vi "Dashboard Main.vi"() -> ()   [LabVIEW 2014]
uses:
  <vilib>/event_ctls.llb/eventvkey.ctl
  <vilib>/Rock Robotics/WPI/Dashboard/WPI_DashboardLogging Global.vi
  <vilib>/Rock Robotics/Network Tables/SD Read Number.vi
  <vilib>/Rock Robotics/Network Tables/SD Read Boolean.vi
  <vilib>/Rock Robotics/Network Tables/SD Write Number.vi
  <vilib>/Rock Robotics/Network Tables/SD Read String.vi
  <vilib>/Utility/config.llb/Write Key (String).vi
  <vilib>/Utility/config.llb/Write Key (I32).vi
  <vilib>/Utility/config.llb/NI_LVConfig.lvlib
panel:
  in  "TCP":refnum<k5>
  in  "Rec Mode":enum32{"Stop", "Record", "Playback"}(radio)
  in  "Vision":u16(ring) items=["Camera Off", "USB Camera SW", "USB Camera HW", "IP Camera"]
  out "Camera IP":string
  out "Image Message":string="Timeout in Camera Communications"
  in  "Dashboard Tab":T1(tab)
  in  "Camera Guide Position":dbl(slide) scale=0.0..320.0
  in  "Camera Settings":T2={"Frame Rate"=30, "Compression"=30, "Size"=1} {"Frame Rate" scale=1.0..30.0; "Size" items=["640x480", "320x240", "160x120"]}
  out "MotorChart R":cluster{"Numeric":dbl, "Numeric":dbl}(graph)
  out "MotorChart L":T3(graph)
  out "MotorSliders R":cluster{"MotorSlide1":dbl, "MotorSlide2":dbl} {"MotorSlide2" scale=-1.0..1.0 scale format="%#_2e"; "MotorSlide1" scale=-1.0..1.0 scale format="%#_2e"}
  out "MotorSliders L":T4 {"MotorSlide4 2" scale=0.0..14.0 scale format="%#_2e"; "MotorSlide2" scale=-1.0..1.0 scale format="%#_2e"; "MotorSlide1" scale=-1.0..1.0 scale format="%#_2e"}
  out "JS1 Z":dbl(slide) scale=-1.0..1.0 scale format="%#_2e"
  out "JS1 Graph":cluster{"X":dbl, "Y":dbl}[](graph)
  out "JS1 Buttons":T5
  out "JS2 Z":dbl(slide) scale=-1.0..1.0 scale format="%#_2e"
  out "JS2 Graph":cluster{"X":dbl, "Y":dbl}[](graph)
  out "JS2 Buttons":T5
  out "Mode":T6(ring)=enum."Auto Disabled"
  in  "DB Camera Config":bool
  out "fps":dbl format="%#.1g"
  out "Mbps":dbl format="%#.1g"
  out "Mbps 2":bool
  out "Current Auto":dbl
  out "Auto/String 3":string caption="DB/String 3"
  out "Auto/String 2":string caption="DB/String 2"
  out "Auto/String 1":string caption="DB/String 1"
  out "Auto/String 0":string caption="Auto"
  out "Can\n  Auto\n  Stack":bool
  out "PID State":T7(ring)
  in  "Training Mode Threshold":dbl=0.8
  out "Drive Mode":bool
  out "Gyro":dbl(knob) scale=0.0..360.0
  in  "Halo Sensitivity":dbl=0.7 min=0.0 max=1.0 step=0.01 format="%.2f"
  out "Encoder Left":dbl
  out "Encoder Right":dbl
  out "Training Enabled":bool
  out "Auto Stack State":T8(ring)
  out "Gripper":bool
  out "Gripper 2":bool
  in  "Test Slider":dbl(slide) scale=0.0..100.0 scale format="%#_3g"
  in  "On/Off":bool caption="Solenoid"
  in  "Test Name":u16(ring) items=["Select the test to run...", "Example Test", "-------------------------------", "List of tests is built in robot code.", "Replace with your own automated tests."]
  in  "Test Tree":string(tree)
  in  "Motor":cluster{"Value":dbl, "Enable":bool} {"Value" scale=-1.0..1.0 scale format="%#_3g"}
  out "Progress":T9 {"Test Progress" scale=0.0..100.0}
  in  "Rev/Fwd":cluster{"Forward":bool, "Reverse":bool}
  in  "Test Ring":u16(ring) items=["Monochrome", "Color"]
  in  "Listbox":i32(listbox)
  out "Tree":string(tree)
  out "Camera Image":T10(plugin-control)
  out "Boolean":bool
  # "Left"
  # "Front"
  # "Right"
  # "Battery"
  # "0 - TOTE+CONTAINER\n1 - DRIVESTRAIGHT FROM STARTING AREA\n2 - DRIVESTRAIGHT FROM VOLDEMORT\n3 - 2 CONTAINER + LEFT TURN\n4 - 2 CONTAINER + RIGHT TURN\n5 - STOP_ALL\n6 - TAPE MEASURE"
  # "Hold BACK button on \nJoystick 1 to switch"
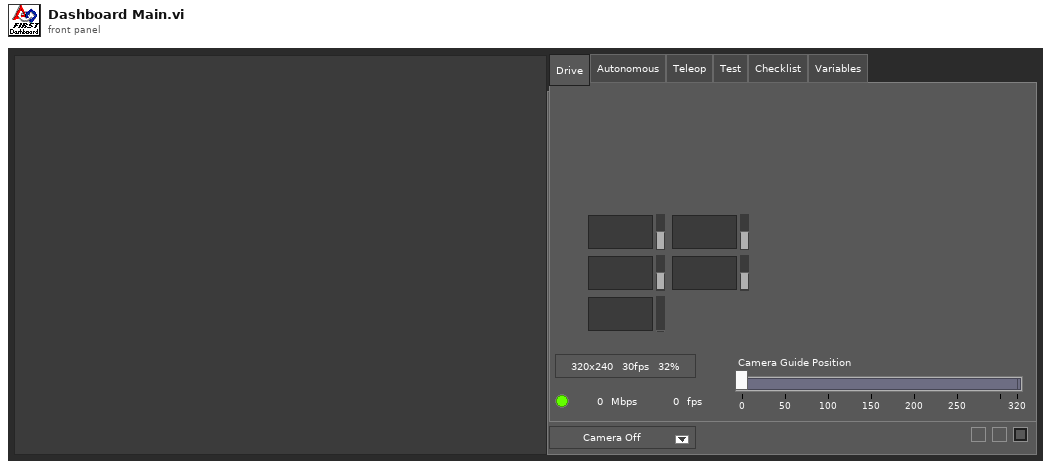
[diagram p1: front panel]
types:
  T1 = enum32{"Drive", "Autonomous", "Teleop", "Test", "Checklist", "Variables"}
  T2 = cluster{"Frame Rate":i32, "Compression":i32, "Size":u16}
  T3 = cluster{"Numeric":dbl, "Numeric":dbl, "Battery V":dbl}
  T4 = cluster{"MotorSlide1":dbl, "MotorSlide2":dbl, "MotorSlide4 2":dbl}
  T5 = cluster{bool, bool, bool, bool, bool, bool, bool, bool, bool, bool, bool, bool}
  T6 = enum8{"Tele-Op Disabled", "Tele-Op Enabled", "Auto Disabled", "Auto Enabled", "Test Disabled", "Test Enabled", "Disconnected", "No Code", "E-Stop"}
  T7 = enum16{"ResetForward", "ResetBack", "PIDControl", "ManualControl", "ZeroEncoderAndTarget", "AutoStack"}
  T8 = enum16{"Disabled", "Initialize", "CalcNewTarget", "Moving", "OpenArm", "CloseArm", "Reset"}
  T9 = cluster{"Test Progress":u8, "Test Progress Text":string}
  T10 = typedef "IMAQ Image.ctl" = refnum<image>
  T11 = enum32{"Drive", "Basic", "Custom", "Test", "Checklist", "Variables"}
  T12 = typedef "Image Type" = u32
  T13 = cluster{"Camera Image":refnum<vi>, "Dashboard Tab":refnum<vi>, "Boolean":refnum<vi>, "Vision":refnum<vi>, "Rec Mode":refnum<vi>, "Test Slider":refnum<vi>, "On/Off ":refnum<vi>, "Test Ring":refnum<vi>, "Rev/Fwd":refnum<vi>, "Test Name":refnum<vi>, "Motor":refnum<vi>, "Progress":refnum<vi>, "CheckList":refnum<vi>, "Tree":refnum<vi>, "Test Tree":refnum<vi>}
  T14 = cluster{"Error Strings":string, "Disable Counts":cluster{u16, u16}, "Rail Faults":cluster{u16, u16, u16}, "Robot IP":string, "DB Mode":u8, "Event Info":cluster{"Name":string, "Type":u8, "Number":u16, "Replay":u8}, "Camera Addr":string}
  T15 = cluster{"Storage":cluster{"Disk Free":u64, "RAM Block":u32, "RAM free":u32}, "CPU Utilization":cluster{"CPU % ISR":sgl, "CPU % Time Crit":sgl, "CPU % Timed Str":sgl, "CPU % High":sgl, "CPU % Above":sgl, "CPU % Normal":sgl, "CPU % Low":sgl}, "CAN":cluster{"% Bus Utilization":sgl, "Bus Off Cnt":u32, "TX_FIFO Full Cnt":u32, "Receive Error Cnt":u8, "Transmit Error Cnt":u8}, "HID":cluster{"HID Outputs":u32, "Rumble Low":u16, "Rumble High":u16}[]}
  T16 = cluster{"Status bits":cluster{"Test Mode":bool, "Autonomous":bool, "Enabled":bool, "Code Start":bool, "Brownout":bool, "Reserved 2":bool, "Reserved 3":bool, "E-Stop":bool}, "Code Trace":cluster{"Disabled":bool, "TeleOp":bool, "Auto":bool, "Test":bool}, "Controller Type":enum16{"unknown", "cRIO", "roboRio"}, "Code?":enum16{"unknown", "noCode", "code"}, "Battery V":dbl}
  T17 = cluster{"Control Bits":cluster{"TestMode":bool, "Autonomous":bool, "Enabled":bool, "FMS Present":bool, bool, bool, bool, "E-Stop":bool}, "Team Station ":u8, "Countdown":sgl, "Joystick Values":cluster{"Axes":dbl[], "Buttons":bool[], "POVs":i16[]}[]}
  T18 = cluster{"Axes":dbl[], "Buttons":bool[], "POVs":i16[]}[]
  T19 = cluster{"Axes":dbl[], "Buttons":bool[], "POVs":i16[]}
  T20 = cluster{"Buttons[0]":bool, "Buttons[1]":bool, "Buttons[2]":bool, "Buttons[3]":bool, "Buttons[4]":bool, "Buttons[5]":bool, "Buttons[6]":bool, "Buttons[7]":bool, "Buttons[8]":bool, "Buttons[9]":bool, "Buttons[10]":bool, "Buttons[11]":bool}
  T21 = typedef "NI_LVConfig.lvlib/Config Data RefNum.ctl" = refnum<k1>
  T22 = cluster{"Operation":enum16{"Update", "Clear"}, "Color Box":u32}[]
  T23 = typedef "eventvkey.ctl" = enum16{"ASCII", "Enter", "Return", "Shift", "Ctrl", "Alt", "Cmd", "Opt", "Caps", "NumLock", "Clear", "Break", "Up", "Down", "Left", "Right", "Insert", "Delete", "Home", "End", "PageUp", "PageDown", "Escape", "Help", "Pause", "ScrollLock", "F1", "F2", "F3", "F4", "F5", "F6", "F7", "F8", "F9", "F10", "F11", "F12", "F13", "F14", "F15", "F16", "F17", "F18", "F19", "F20", "F21", "F22", "F23", "F24", "Play", "VolumeUp", "VolumeDown", "Mute", "Two Byte Char"}
  T24 = cluster{"Image Size":bool, "Image Type":bool, "Pixel Value":bool, "ROI Information":bool, "Zoom Factor":bool}
  T25 = enum8{"Enabled", "Disabled", "Disabled and Grayed Out"}
  T26 = cluster{"Operation":enum16{"Update", "Clear"}, "Color Box":u32}
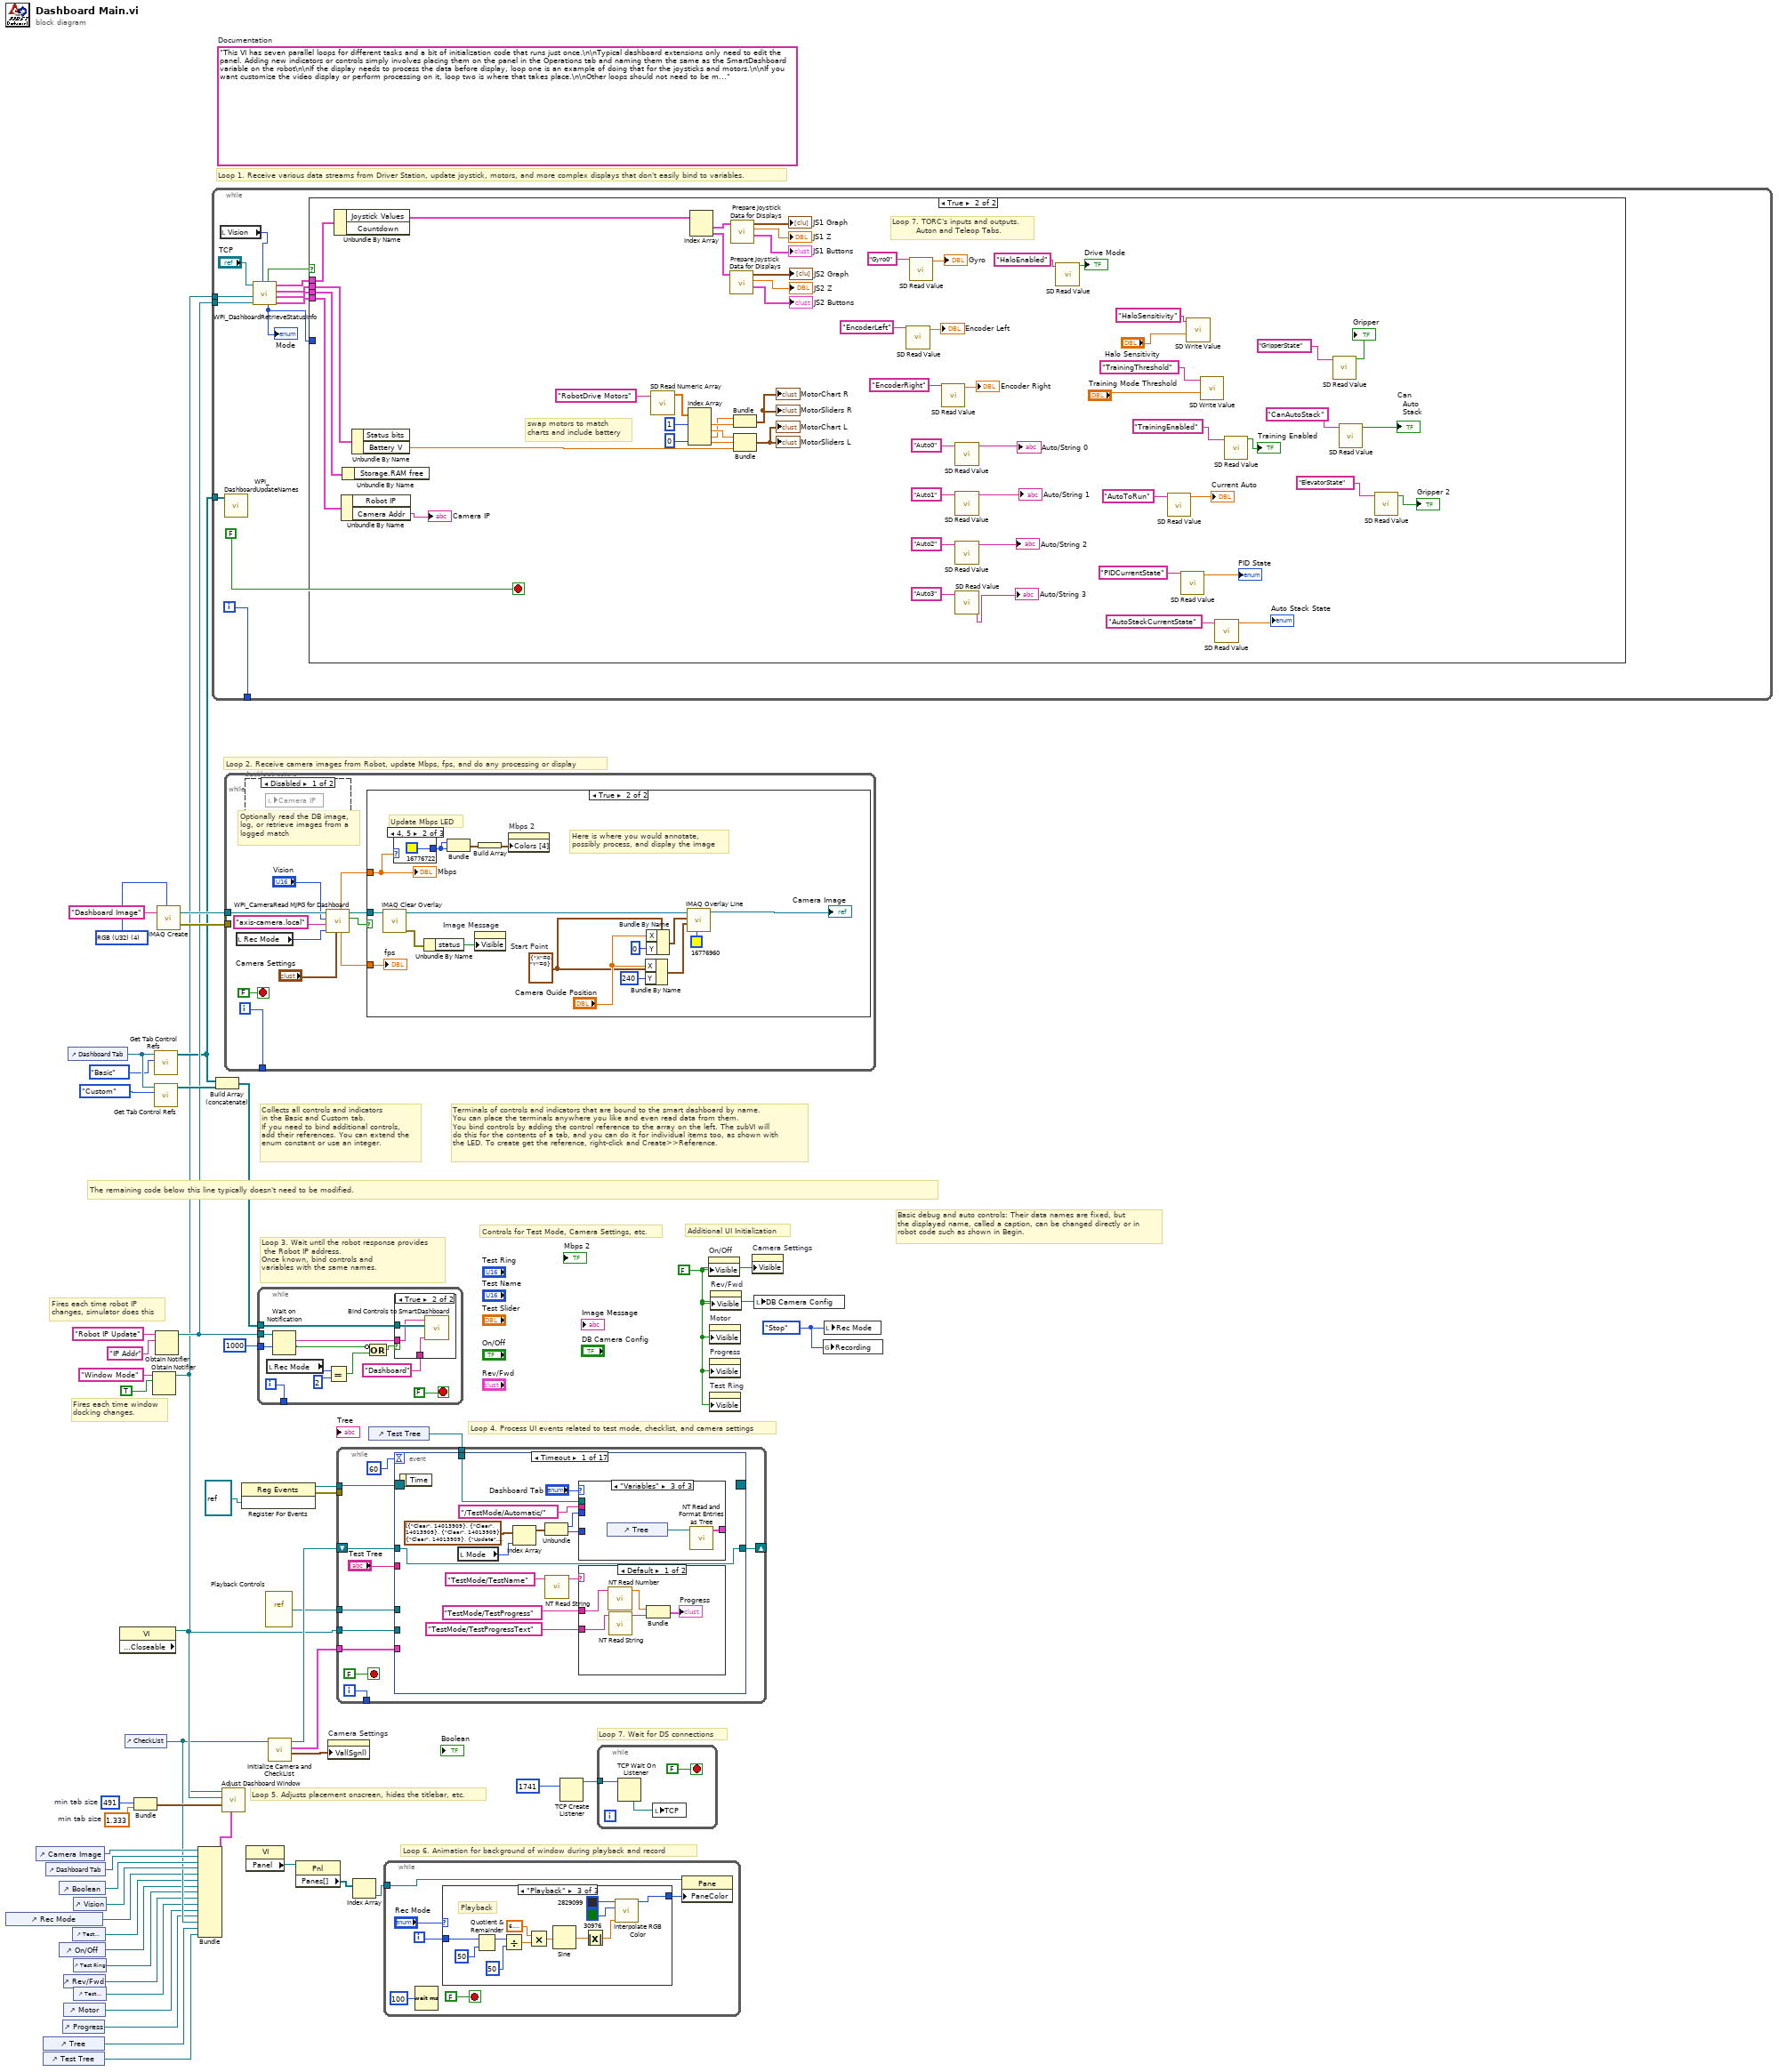
[diagram p0: block diagram]
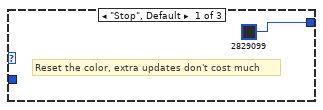
[diagram p3: hidden frame]
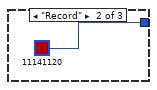
[diagram p4: hidden frame]
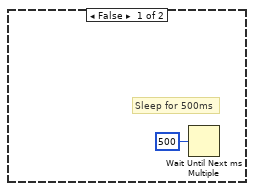
[diagram p7: hidden frame]
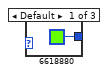
[diagram p8: hidden frame]
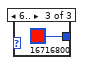
[diagram p9: hidden frame]
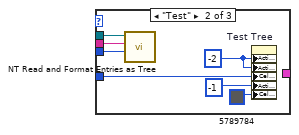
[diagram p11: hidden frame]
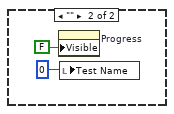
[diagram p12: hidden frame]
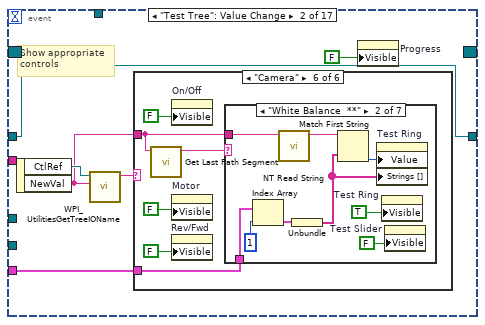
[diagram p13: hidden frame]
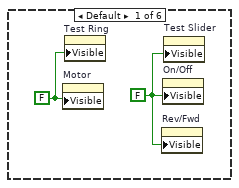
[diagram p14: hidden frame]
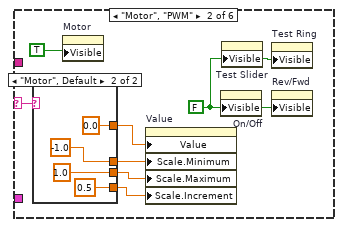
[diagram p15: hidden frame]
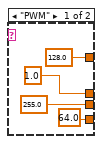
[diagram p16: hidden frame]
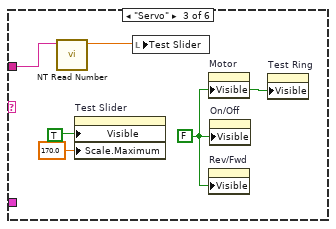
[diagram p17: hidden frame]
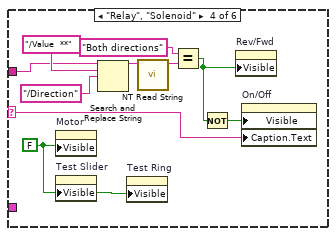
[diagram p18: hidden frame]
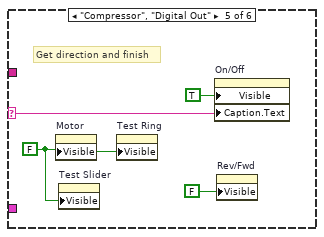
[diagram p19: hidden frame]
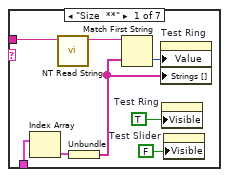
[diagram p20: hidden frame]
diagram:
  w24 = 491  # min tab size
  w23 = 1.333  # min tab size
  w32 = enum32{"Stop", "Record", "Playback"}."Stop" ("Rec Mode")
  w6 = FALSE ("Visible")
  (unwired) "This VI has seven parallel loops for different tasks and a bit of initialization code that runs just once.\n\nTypical dashboard extensions only need to edit the panel. Adding new indicators or controls simply involves placing them on the panel in the Operations tab and naming them the same as the SmartDashboard variable on the robot\n\nIf the display needs to process the data before display, loop one is an example of doing that for the joysticks and motors.\n\nIf you want customize the video display or perform processing on it, loop two is where that takes place.\n\nOther loops should not need to be modified. They are pretty standard, and document the task they perform."  # Documentation
  w52 = T12 4 items=["Grayscale (U8)", "Grayscale (I16)", "Grayscale (SGL)", "Complex (CSG)", "RGB (U32)", "HSL (U32)", "RGB (U64)"] ("Image Type")
  # "Loop 7. Wait for DS connections"
  # "Basic debug and auto controls: Their data names are fixed, but\nthe displayed name, called a caption, can be changed directly or in\nrobot code such as shown in Begin."
  # "Controls for Test Mode, Camera Settings, etc."
  # "Additional UI Initialization"
  # "Loop 6. Animation for background of window during playback and record"
  # "Fires each time robot IP\nchanges, simulator does this"
  # "Fires each time window\ndocking changes."
  # "Collects all controls and indicators\nin the Basic and Custom tab.\nIf you need to bind additional controls,\nadd their references. You can extend the\nenum constant or use an integer."
  # "The remaining code below this line typically doesn't need to be modified."
  # "Loop 4. Process UI events related to test mode, checklist, and camera settings"
  # "Terminals of controls and indicators that are bound to the smart dashboard by name.\nYou can place the terminals anywhere you like and even read data from them.\nYou bind controls by adding the control reference to the array on the left. The subVI will\ndo this for the contents of a tab, and you can do it for individual items too, as shown with\nthe LED. To create get the reference, right-click and Create>>Reference."
  # "Loop 3. Wait until the robot response provides\n the Robot IP address.\nOnce known, bind controls and\nvariables with the same names."
  # "Loop 5. Adjusts placement onscreen, hides the titlebar, etc."
  # "Loop 1. Receive various data streams from Driver Station, update joystick, motors, and more complex displays that don't easily bind to variables."
  # "Loop 2. Receive camera images from Robot, update Mbps, fps, and do any processing or display"
  n1 = control-ref of="Rec Mode"() -> (w12:refnum<vi>)
  n2 = control-ref of="Camera Image"() -> (w27:refnum<vi>)
  n3 = control-ref of="Tree"() -> (w16:refnum<vi>)
  n4 = control-ref of="Test Tree"() -> (w15:refnum<vi>)
  n5 = control-ref of="Dashboard Tab"() -> (w26:refnum<vi>)
  n6 = control-ref of="Boolean"() -> (w21:refnum<vi>)
  n7 = control-ref of="On/Off"() -> (w10:refnum<vi>)
  n8 = control-ref of="Progress"() -> (w7:refnum<vi>)
  n9 = control-ref of="Rev/Fwd"() -> (w8:refnum<vi>)
  n10 = control-ref of="Motor"() -> (w13:refnum<vi>)
  n11 = control-ref of="Dashboard Tab"() -> (w30:refnum<vi>)
  n12 = control-ref of="Test Slider"() -> (w11:refnum<vi>)
  n13 = control-ref of="Vision"() -> (w25:refnum<vi>)
  n14 = control-ref of="Test Ring"() -> (w9:refnum<vi>)
  n15 = control-ref of="Test Name"() -> (w14:refnum<vi>)
  n16 = property class="VI" props=["Front Panel.Closeable"]() -> (reference out=w31:refnum<vi>)  [unwired: 2 in, 2 out]
  n17 = control-ref of="CheckList"() -> (w17:refnum<vi>)
  n18 = Bundle("min tab size"=w24, "min tab size"=w23) -> (w22:cluster{"min tab size":i32, "min tab size":dbl})  [unwired: 1 in]
  n19 = Obtain Notifier(name (unnamed)="Window Mode", notification data type=TRUE) -> (notifier out=w3:refnum<notifier>)  [unwired: 2 in, 2 out]
  n20 = call <vilib>:"Get Tab Control Refs.vi"("Page Index"=T11."Basic" ("Dashboard Tab"), "TabControl in"=w30) -> ("ControlsOnPage"=w4:refnum<vi>[])  [unwired: 9 in]
  n21 = call <vilib>:"Get Tab Control Refs.vi"("Page Index"=T11."Custom" ("Dashboard Tab"), "TabControl in"=w30) -> ("ControlsOnPage"=w29:refnum<vi>[])  [unwired: 9 in]
  n22 = Obtain Notifier(name (unnamed)="Robot IP Update", notification data type="IP Addr" ("name (unnamed)")) -> (notifier out=w5:refnum<notifier>)  [unwired: 2 in, 2 out]
  n23 = call "IMAQ Create"("Image Name"="Dashboard Image", "Image Type"=w52) -> ("New Image"=w50:T10, "error out"=w49:errorcluster)  [unwired: 2 in, 1 out]
  n24 = Bundle("Camera Image"=w27, "Dashboard Tab"=w26, "Boolean"=w21, "Vision"=w25, "Rec Mode"=w12, "Test Slider"=w11, "On/Off"=w10, "Test Ring"=w9, "Rev/Fwd"=w8, "Test Name"=w14, "Motor"=w13, "Progress"=w7, "CheckList"=w17, "Tree"=w16, "Test Tree"=w15) -> (w18:T13)  [unwired: 1 in]
  n25 = while {
    tunnel: [w64] -> _
    tunnel: w5 -> [w63]
    tunnel: w4 -> [w62]
    tunnel: w3 -> [w59]
    i -> [w64]
    stop <- FALSE stop-if-true
    n26 = local read "Vision"() -> (w61:u16)
    n27 = call <vilib>:"WPI_DashboardUpdateNames.vi"("Controls on Tab"=w62) -> ()  [unwired: 11 in]
    n28 = call <vilib>:"WPI_DashboardRetrieveStatusInfo.vi"("Vision"=w61, "Binding Refnum"=w63, "Window Mode Notifier"=w59, "TCP Cnx"="TCP") -> ("Power and Errors"=w55:T14, "Robot Metrics"=w56:T15, "Status Info"=w57:T16, "Control Info"=w58:T17, "Robot Mode"=w54:T6, "Process?"=w53:bool)  [unwired: 2 in]
    "Mode" <- w54
    n29 = case shown="True" w53 {
      tunnel: w57 -> [_ w124]
      tunnel: w56 -> [_ w123]
      tunnel: w58 -> [_ w122]
      tunnel: w55 -> [_ w121]
      tunnel: w54 -> [_ _]
      frame False {
      }
      frame True {
        # "Loop 7. TORC's inputs and outputs.\n         Auton and Teleop Tabs."
        # "swap motors to match\ncharts and include battery"
        n30 = Unbundle By Name(w122) -> ("Joystick Values"=w109:T18)  [unwired: 1 out]
        n31 = Unbundle By Name(w121) -> ("Camera Addr"=→"Camera IP":string)  [unwired: 1 out]
        n32 = Unbundle By Name(w123) -> ()  [unwired: 1 out]
        n33 = Unbundle By Name(w124) -> ("Battery V"=w110:dbl)  [unwired: 1 out]
        n34 = call <vilib>:"SD Read Numeric Array.vi"("Name"="RobotDrive Motors") -> ("Numeric Array"=w112:dbl[])  [unwired: 8 in, 2 out]
        n35 = Index Array(array=w112, index #1=1, index #4=0) -> (element #1=w116:dbl, element #2=w117:dbl, element #3=w115:dbl, element #4=w120:dbl)  [unwired: 2 in]
        n36 = Index Array(array=w109) -> (element #1=w108:T19, element #2=w103:T19)  [unwired: 2 in]
        n37 = call "Prepare Joystick Data for Displays.vi"("Joystick Values"=w103) -> ("Buttons"=→"JS2 Buttons":T20, "Z Axis"=→"JS2 Z":dbl, "Cartesian Data"=→"JS2 Graph":cluster{"X axis":dbl, "X axis":dbl}[])  [unwired: 8 in]
        n38 = call "Prepare Joystick Data for Displays.vi"("Joystick Values"=w108) -> ("Buttons"=→"JS1 Buttons":T20, "Z Axis"=→"JS1 Z":dbl, "Cartesian Data"=→"JS1 Graph":cluster{"X axis":dbl, "X axis":dbl}[])  [unwired: 8 in]
        n39 = Bundle("Numeric"=w115, "Numeric"=w116) -> (→"MotorChart R" →"MotorSliders R":cluster{"Numeric":dbl, "Numeric":dbl})  [unwired: 1 in]
        n40 = Bundle("Numeric"=w117, "Numeric"=w120, "Battery V"=w110) -> (→"MotorChart L" →"MotorSliders L":T3)  [unwired: 1 in]
        n41 = call-poly <vilib>:"SD Read Value.vi"("Name"="EncoderLeft") -> ("Numeric"=→"Encoder Left":dbl)  [unwired: 8 in, 2 out]
        n42 = call-poly <vilib>:"SD Read Value.vi"("Name"="Gyro0") -> ("Numeric"=→"Gyro":dbl)  [unwired: 8 in, 2 out]
        n43 = call-poly <vilib>:"SD Read Value.vi"("Name"="EncoderRight") -> ("Numeric"=→"Encoder Right":dbl)  [unwired: 8 in, 2 out]
        n44 = call-poly <vilib>:"SD Read Value.vi"("Name"="Auto0") -> ("String"=→"Auto/String 0":string)  [unwired: 8 in, 2 out]
        n45 = call-poly <vilib>:"SD Read Value.vi"("Name"="Auto1") -> ("String"=→"Auto/String 1":string)  [unwired: 8 in, 2 out]
        n46 = call-poly <vilib>:"SD Read Value.vi"("Name"="Auto2") -> ("String"=→"Auto/String 2":string)  [unwired: 8 in, 2 out]
        n47 = call-poly <vilib>:"SD Read Value.vi"("Name"="Auto3") -> ("String"=→"Auto/String 3":string)  [unwired: 8 in, 2 out]
        n48 = call-poly <vilib>:"SD Read Value.vi"("Name"="HaloEnabled") -> ("Boolean"=→"Drive Mode":bool)  [unwired: 8 in, 2 out]
        n49 = call-poly <vilib>:"SD Read Value.vi"("Name"="AutoToRun") -> ("Numeric"=→"Current Auto":dbl)  [unwired: 8 in, 2 out]
        n50 = call-poly <vilib>:"SD Read Value.vi"("Name"="PIDCurrentState") -> ("Numeric"=→"PID State":dbl)  [unwired: 8 in, 2 out]
        n51 = call-poly <vilib>:"SD Write Value.vi"("Numeric"="Halo Sensitivity", "Name"="HaloSensitivity") -> ()  [unwired: 8 in, 2 out]
        n52 = call-poly <vilib>:"SD Write Value.vi"("Numeric"="Training Mode Threshold", "Name"="TrainingThreshold") -> ()  [unwired: 8 in, 2 out]
        n53 = call-poly <vilib>:"SD Read Value.vi"("Name"="AutoStackCurrentState") -> ("Numeric"=→"Auto Stack State":dbl)  [unwired: 8 in, 2 out]
        n54 = call-poly <vilib>:"SD Read Value.vi"("Name"="TrainingEnabled") -> ("Boolean"=→"Training Enabled":bool)  [unwired: 8 in, 2 out]
        n55 = call-poly <vilib>:"SD Read Value.vi"("Name"="GripperState") -> ("Boolean"=→"Gripper":bool)  [unwired: 8 in, 2 out]
        n56 = call-poly <vilib>:"SD Read Value.vi"("Name"="CanAutoStack") -> ("Boolean"=→"Can\n  Auto\n  Stack":bool)  [unwired: 8 in, 2 out]
        n57 = call-poly <vilib>:"SD Read Value.vi"("Name"="ElevatorState") -> ("Boolean"=→"Gripper 2":bool)  [unwired: 8 in, 2 out]
      }
    }
  }
  n58 = Build Array (concatenate)(w4, w29) -> (w28:refnum<vi>[])
  n59 = call "Adjust Dashboard Window.vi"("Sizing Refnums"=w18, "Size Constraints"=w22, "VI"=w31, "Notifier in"=w3) -> ()  [unwired: 8 in]
  n60 = while {
    tunnel: w50 -> [w133]
    tunnel: w49 -> [_]
    tunnel: [w134] -> _
    i -> [w134]
    stop <- FALSE stop-if-true
    # "Optionally read the DB image,\nlog, or retrieve images from a\nlogged match"
    n61 = local read "Rec Mode"() -> (w127:enum32{"Stop", "Record", "Playback"})
    n62 = disable-structure shown="Disabled" {
      frame Disabled {
        n63 = local read "Camera IP"() -> ()  [unwired: 1 in]
      }
      frame Enabled {
      }
    }
    n64 = call <vilib>:"WPI_CameraRead MJPG for Dashboard.vi"("Camera Settings"="Camera Settings", "Rec Mode"=w127, "Camera IP"="axis-camera.local" ("Name"), "Camera Mode"="Vision", "Refnum in"=w133) -> ("Active"=w131:bool, "Refnum out"=w132:T10, "FPS"=w130:dbl, "Bandwidth (Mbps)"=w129:dbl)  [unwired: 3 in]
    n65 = case shown="True" w131 {
      tunnel: w132 -> [_ w148]
      tunnel: w129 -> [_ w147]
      tunnel: w130 -> [_ w146]
      frame False {
        # "Sleep for 500ms"
        n66 = Wait Until Next ms Multiple(millisecond multiple=u32 500) -> ()  [unwired: 1 out]
      }
      frame True {
        w139 = cluster{"X":i32, "Y":i32} {"X"=0, "Y"=0}  # Start Point
        # "Here is where you would annotate,\npossibly process, and display the image"
        # "Update Mbps LED"
        n67 = call "IMAQ Clear Overlay"("Image"=w148) -> ("error out"=w152:errorcluster, "Image Out"=w145:T10)  [unwired: 2 in, 7 out]
        n68 = case shown="4, 5" w147 {
          tunnel: [u32 6618880 ("Color Box") u32 16776722 ("Color Box") u32 16716800 ("Color Box")] -> w149
          frame Default {
          }
          frame 4, 5 {
          }
          frame 6.. {
          }
        }
        n69 = Unbundle By Name(w152) -> ("status"=w153:bool)
        n70 = Bundle("Color Box"=w149, "Color Box"=w149) -> (w151:cluster{"Color Box":u32, "Color Box":u32})  [unwired: 1 out]
        n71 = property on="Image Message" class="Str"("Visible"=w153) -> ()  [unwired: 2 in, 2 out]
        n72 = Build Array(w151) -> (w150:cluster{"Color Box":u32, "Color Box":u32}[])
        n73 = property on="Mbps 2" class="Bool (strict)"("Colors [4]"=w150) -> ()  [unwired: 2 in, 2 out]
        n74 = Bundle By Name(cluster=w139, "X"="Camera Guide Position", "Y"=240) -> (w138:cluster{"X":i32, "Y":i32})
        n75 = Bundle By Name(cluster=w139, "X"="Camera Guide Position", "Y"=0) -> (w143:cluster{"X":i32, "Y":i32})
        n76 = call "IMAQ Overlay Line"("Color"=u32 16776960, "End Point"=w138, "Start Point"=w143, "Image"=w145) -> ("Image Out"=→"Camera Image":T10)  [unwired: 6 in, 1 out]
        "Mbps" <- w147
        "fps" <- w146
      }
    }
  }
  n77 = register-events(refnum<vi> refnum) -> (reference out=w36:refnum<event-registration>, error out=w35:errorcluster)  [unwired: 2 in]
  n78 = property class="VI"() -> ("Panel"=w39:refnum<vi>)  [unwired: 2 in, 2 out]
  n79 = while {
    tunnel: w28 -> [w168]
    tunnel: w5 -> [w166]
    tunnel: [w164] -> _
    tunnel: u32 1000 ("milliseconds to wait") -> [w163]
    i -> [w164]
    stop <- FALSE stop-if-true
    n80 = local read "Rec Mode"() -> (w159:enum32{"Stop", "Record", "Playback"})
    n81 = Wait on Notification(notifier=w166, timeout in ms (-1)=w163) -> (notification=w165:string, timed out?=w161:bool)  [unwired: 2 in, 2 out]
    n82 = Equal?(x=w159, y=u16 2 ("Rec Mode")) -> (x = y?=w160:bool)
    n83 = Compound Arithmetic op=OR(invert w161, w160) -> (w162:bool)
    n84 = case shown="True" w162 {
      tunnel: w168 -> [_ w171]
      tunnel: w165 -> [_ w170]
      tunnel: "Dashboard" -> [_ w169]
      frame False {
      }
      frame True {
        n85 = call <vilib>:"Bind Controls to SmartDashboard.vi"("Client Name"=w169, "Bound Control Refs"=w171, "Server IP Address"=w170) -> ()  [unwired: 9 in]
      }
    }
  }
  n86 = vi-ref "Playback Controls.vi"() -> (w37:refnum<vi>)
  n87 = call "Initialize Camera and CheckList.vi"("ListBox in"=w17) -> ("Cluster"=w43:cluster{"value":i32, "value":i32, "index":i32}, "Array"=w44:cluster{string[]}[], "File Refnum"=w42:T21)  [unwired: 8 in]
  n88 = property class="Pnl"(reference=w39) -> ("Panes[]"=w40:refnum<vi>[])  [unwired: 1 in, 2 out]
  n89 = property on="Camera Settings" class="Clust (strict)"("Val(Sgnl)"=w43) -> ()  [unwired: 2 in, 2 out]
  n90 = Index Array(array=w40) -> (element=w38:refnum<vi>)  [unwired: 1 in]
  n91 = control-ref of="Test Tree"() -> (w41:refnum<vi>)
  n92 = while {
    tunnel: w44 -> [w179]
    shift-right: [w178] -> _
    shift-left: w42 -> [w177]
    tunnel: [w176] -> _
    tunnel: w41 -> [w175]
    tunnel: w37 -> [w174]
    tunnel: w36 -> [w173]
    tunnel: w35 -> [_]
    tunnel: w31 -> [w172]
    i -> [w176]
    stop <- FALSE stop-if-true
    n93 = event shown="[0] Timeout" {
      selector: w173 -> [_ _ _ _ _ _ _ _ _ _ _ _ _ _ _ _ _]
      dyn-events: [_ _ _ _ _ _ _ _ _ _ _ _ _ w417 _ _ _] -> _
      timeout: u32 60 ("milliseconds to wait") -> [_ _ _ _ _ _ _ _ _ _ _ _ _ _ _ _ _]
      tunnel: w175 -> [w191 _ _ _ _ _ _ _ _ _ _ _ _ _ _ _ _]
      tunnel: "Test Tree" -> [_ _ _ _ _ _ _ _ w386 w394 w396 w400 w408 _ _ _ _]
      tunnel: w179 -> [_ w213 _ _ _ _ w350 w380 _ _ _ _ _ _ _ _ _]
      tunnel: [w187 w212 w311 w316 w324 w336 w349 w373 w385 w392 w395 w399 w407 w419 w433 w434 w444] -> w178
      tunnel: w177 -> [w187 w212 w311 w316 w324 w336 w348 w373 w385 w392 w395 w399 w407 w419 w433 w434 w444]
      tunnel: w174 -> [_ _ _ _ _ _ _ _ _ _ _ _ _ w420 _ w437 _]
      tunnel: w172 -> [_ _ _ _ _ _ _ _ _ _ _ _ _ w415 _ _ _]
      event Timeout {
        n94 = event-data() -> ()  [unwired: 1 in, 1 out]
        n95 = local read "Mode"() -> (w190:T6)
        n96 = Index Array(array=T22 [{"Operation"=enum."Clear", "Color Box"=14013909}, {"Operation"=enum."Clear", "Color Box"=14013909}, {"Operation"=enum."Clear", "Color Box"=14013909}, {"Operation"=enum."Clear", "Color Box"=14013909}, {"Operation"=enum."Update", "Color Box"=14013909}, {"Operation"=enum."Update", "Color Box"=16777215}, {"Operation"=enum."Clear", "Color Box"=14013909}, {"Operation"=enum."Clear", "Color Box"=14013909}, {"Operation"=enum."Clear", "Color Box"=14013909}], index=w190) -> (element=w185:T26)
        n97 = Unbundle(w185) -> ("Operation"=w184:enum16{"Update", "Clear"}, "Color Box"=w183:u32)
        n98 = call <vilib>:"NT Read String.vi"("Name"="TestMode/TestName") -> ("String"=w194:string)  [unwired: 9 in, 1 out]
        n99 = case shown="\"Variables\"" "Dashboard Tab" {
          tunnel: w191 -> [_ w202 _]
          tunnel: "/TestMode/Automatic/" ("Name Pattern") -> [_ w201 _]
          tunnel: w184 -> [_ w200 _]
          tunnel: [_ _ w204] -> _
          tunnel: w183 -> [_ w196 _]
          frame "Teleop", Default {
          }
          frame "Test" {
            w199 = -2 ("Active Item:Row Number")
            n100 = call <vilib>:"NT Read and Format Entries as Tree.vi"("Operation"=w200, "Name Pattern"=w201, "Tree Refnum"=w202) -> ()  [unwired: 7 in, 2 out]
            n101 = property on="Test Tree" class="Tree (strict)"("Active Item Row Number"=w199, "ActiveColNum"=w199, "CellBG"=w196, "Active Item Row Number"=-1 ("Active Item:Row Number"), "CellBG"=u32 5789784 ("Color Box")) -> ()  [unwired: 2 in, 2 out]
          }
          frame "Variables" {
            n102 = control-ref of="Tree"() -> (w203:refnum<vi>)
            n103 = call <vilib>:"NT Read and Format Entries as Tree.vi"("Tree Refnum"=w203) -> ("Formatted Strings"=w204:cluster{"Name":string, "Value":string}[])  [unwired: 9 in, 1 out]
          }
        }
        n104 = case shown="Default" w194 {
          tunnel: "TestMode/TestProgress" ("Name") -> [w206 _]
          tunnel: "TestMode/TestProgressText" ("Name") -> [w205 _]
          frame Default {
            n105 = call <vilib>:"NT Read Number.vi"("Name"=w206) -> ("Numeric"=w207:dbl)  [unwired: 9 in, 1 out]
            n106 = call <vilib>:"NT Read String.vi"("Name"=w205) -> ("String"=w208:string)  [unwired: 9 in, 1 out]
            n107 = Bundle("Numeric"=w207, "String"=w208) -> (→"Progress":cluster{"Numeric":dbl, "String":string})  [unwired: 1 in]
          }
          frame "" {
            n108 = property on="Progress" class="Clust (strict)"("Visible"=FALSE) -> ()  [unwired: 2 in, 2 out]
            n109 = local write "Test Name"(u16 0) -> ()
          }
        }
      }
      event "Test Tree": Value Change {
        # "Show appropriate\ncontrols"
        n110 = event-data() -> ("CtlRef"=w216:refnum<vi>, "NewVal"=w214:string)  [unwired: 1 in]
        n111 = call <vilib>:"WPI_UtilitiesGetTreeIOName.vi"("NewVal"=w214, "TreeControl in"=w216) -> ("I/O Name"=w217:string)  [unwired: 9 in]
        n112 = case shown="\"Camera\"" w217 {
          selector: w217 -> [_ w224 _ w242 w251 _]
          tunnel: w214 -> [_ _ w239 w241 _ w258]
          tunnel: w213 -> [_ _ _ _ _ w257]
          frame Default {
            w219 = FALSE ("Visible")
            w218 = FALSE ("Visible")
            n113 = property on="Motor" class="Clust (strict)"("Visible"=w218) -> ()  [unwired: 2 in, 2 out]
            n114 = property on="Test Ring" class="Ring (strict)"("Visible"=w218) -> ()  [unwired: 2 in, 2 out]
            n115 = property on="Rev/Fwd" class="Clust (strict)"("Visible"=w219) -> ()  [unwired: 2 in, 2 out]
            n116 = property on="On/Off" class="Bool (strict)"("Visible"=w219) -> ()  [unwired: 2 in, 2 out]
            n117 = property on="Test Slider" class="Slide (strict)"("Visible"=w219) -> ()  [unwired: 2 in, 2 out]
          }
          frame "Motor", "PWM" {
            w225 = FALSE ("Visible")
            n118 = case shown="\"Motor\", Default" w224 {
              tunnel: [1.0 ("Value") -1.0 ("Value")] -> w223
              tunnel: [255.0 ("Value") 1.0 ("Value")] -> w222
              tunnel: [128.0 ("Value") 0.0 ("Value")] -> w221
              tunnel: [64.0 ("Value") 0.5 ("Value")] -> w220
              frame "PWM" {
              }
              frame "Motor", Default {
              }
            }
            n119 = property on="Motor" class="Clust (strict)"("Visible"=TRUE) -> ()  [unwired: 2 in, 2 out]
            n120 = property on="Value" class="Slide (strict)"("Value"=w221, "Scale.Minimum"=w223, "Scale.Maximum"=w222, "Scale.Increment"=w220) -> ()  [unwired: 2 in, 2 out]
            n121 = property on="On/Off" class="Bool (strict)"("Visible"=w225) -> ()  [unwired: 2 in, 2 out]
            n122 = property on="Test Slider" class="Slide (strict)"("Visible"=w225) -> ()  [unwired: 2 in, 2 out]
            n123 = property on="Test Ring" class="Ring (strict)"("Visible"=w225) -> ()  [unwired: 2 in, 2 out]
            n124 = property on="Rev/Fwd" class="Clust (strict)"("Visible"=w225) -> ()  [unwired: 2 in, 2 out]
          }
          frame "Servo" {
            w237 = FALSE ("Visible")
            n125 = call <vilib>:"NT Read Number.vi"("Name"=w239) -> ("Numeric"=w238:dbl)  [unwired: 9 in, 1 out]
            n126 = property on="Test Slider" class="Slide (strict)"("Visible"=TRUE, "Scale.Maximum"=170.0 ("Scale.Range:Maximum")) -> ()  [unwired: 2 in, 2 out]
            n127 = local write "Test Slider"(w238) -> ()
            n128 = property on="Motor" class="Clust (strict)"("Visible"=w237) -> ()  [unwired: 2 in, 2 out]
            n129 = property on="Rev/Fwd" class="Clust (strict)"("Visible"=w237) -> ()  [unwired: 2 in, 2 out]
            n130 = property on="On/Off" class="Bool (strict)"("Visible"=w237) -> ()  [unwired: 2 in, 2 out]
            n131 = property on="Test Ring" class="Ring (strict)"("Visible"=w237) -> ()  [unwired: 2 in, 2 out]
          }
          frame "Relay", "Solenoid" {
            w240 = FALSE ("Visible")
            n132 = property on="Motor" class="Clust (strict)"("Visible"=w240) -> ()  [unwired: 2 in, 2 out]
            n133 = property on="Test Slider" class="Slide (strict)"("Visible"=w240) -> ()  [unwired: 2 in, 2 out]
            n134 = Search and Replace String(input string=w241, search string="/Value  **", replace string="/Direction") -> (result string=w247:string)  [unwired: 5 in, 3 out]
            n135 = property on="Test Ring" class="Ring (strict)"("Visible"=w240) -> ()  [unwired: 2 in, 2 out]
            n136 = call <vilib>:"NT Read String.vi"("Name"=w247) -> ("String"=w245:string)  [unwired: 9 in, 1 out]
            n137 = Equal?(x="Both directions", y=w245) -> (x = y?=w243:bool)
            n138 = Not(x=w243) -> (.not. x?=w244:bool)
            n139 = property on="Rev/Fwd" class="Clust (strict)"("Visible"=w243) -> ()  [unwired: 2 in, 2 out]
            n140 = property on="On/Off" class="Bool (strict)"("Visible"=w244, "Caption.Text"=w242) -> ()  [unwired: 2 in, 2 out]
          }
          frame "Compressor", "Digital Out" {
            w250 = FALSE ("Visible")
            # "Get direction and finish"
            n141 = property on="Motor" class="Clust (strict)"("Visible"=w250) -> ()  [unwired: 2 in, 2 out]
            n142 = property on="Test Slider" class="Slide (strict)"("Visible"=w250) -> ()  [unwired: 2 in, 2 out]
            n143 = property on="Test Ring" class="Ring (strict)"("Visible"=w250) -> ()  [unwired: 2 in, 2 out]
            n144 = property on="On/Off" class="Bool (strict)"("Visible"=TRUE, "Caption.Text"=w251) -> ()  [unwired: 2 in, 2 out]
            n145 = property on="Rev/Fwd" class="Clust (strict)"("Visible"=FALSE) -> ()  [unwired: 2 in, 2 out]
          }
          frame "Camera" {
            n146 = call <vilib>:"Get Last Path Segment.vi"("String in"=w258) -> ("String out"=w259:string)  [unwired: 10 in]
            n147 = property on="On/Off" class="Bool (strict)"("Visible"=FALSE) -> ()  [unwired: 2 in, 2 out]
            n148 = property on="Motor" class="Clust (strict)"("Visible"=FALSE) -> ()  [unwired: 2 in, 2 out]
            n149 = property on="Rev/Fwd" class="Clust (strict)"("Visible"=FALSE) -> ()  [unwired: 2 in, 2 out]
            n150 = case shown="\"White Balance  **\"" w259 {
              tunnel: w258 -> [w265 w274 w283 w292 w301 _ w307]
              tunnel: w257 -> [w263 w271 w280 w289 w298 _ _]
              frame "Size  **" {
                n151 = Index Array(array=w263) -> (element=w262:cluster{string[]})  [unwired: 1 in]
                n152 = call <vilib>:"NT Read String.vi"("Name"=w265) -> ("String"=w264:string)  [unwired: 9 in, 1 out]
                n153 = Unbundle(w262) -> (w260:string[])
                n154 = Match First String(2:w260, 3:w264) -> (0:w261:i32)  [unwired: 1 out]
                n155 = property on="Test Ring" class="Ring (strict)"("Value"=w261, "Strings []"=w260) -> ()  [unwired: 2 in, 2 out]
                n156 = property on="Test Ring" class="Ring (strict)"("Visible"=TRUE) -> ()  [unwired: 2 in, 2 out]
                n157 = property on="Test Slider" class="Slide (strict)"("Visible"=FALSE) -> ()  [unwired: 2 in, 2 out]
              }
              frame "White Balance  **" {
                n158 = Index Array(array=w271, index=1) -> (element=w272:cluster{string[]})
                n159 = call <vilib>:"NT Read String.vi"("Name"=w274) -> ("String"=w273:string)  [unwired: 9 in, 1 out]
                n160 = Unbundle(w272) -> (w269:string[])
                n161 = Match First String(2:w269, 3:w273) -> (0:w268:i32)  [unwired: 1 out]
                n162 = property on="Test Ring" class="Ring (strict)"("Value"=w268, "Strings []"=w269) -> ()  [unwired: 2 in, 2 out]
                n163 = property on="Test Ring" class="Ring (strict)"("Visible"=TRUE) -> ()  [unwired: 2 in, 2 out]
                n164 = property on="Test Slider" class="Slide (strict)"("Visible"=FALSE) -> ()  [unwired: 2 in, 2 out]
              }
              frame "Exposure  **" {
                n165 = Index Array(array=w280, index=2) -> (element=w281:cluster{string[]})
                n166 = call <vilib>:"NT Read String.vi"("Name"=w283) -> ("String"=w282:string)  [unwired: 9 in, 1 out]
                n167 = Unbundle(w281) -> (w277:string[])
                n168 = Match First String(2:w277, 3:w282) -> (0:w278:i32)  [unwired: 1 out]
                n169 = property on="Test Ring" class="Ring (strict)"("Value"=w278, "Strings []"=w277) -> ()  [unwired: 2 in, 2 out]
                n170 = property on="Test Ring" class="Ring (strict)"("Visible"=TRUE) -> ()  [unwired: 2 in, 2 out]
                n171 = property on="Test Slider" class="Slide (strict)"("Visible"=FALSE) -> ()  [unwired: 2 in, 2 out]
              }
              frame "Exposure Priority  **" {
                n172 = Index Array(array=w289, index=3) -> (element=w290:cluster{string[]})
                n173 = call <vilib>:"NT Read String.vi"("Name"=w292) -> ("String"=w291:string)  [unwired: 9 in, 1 out]
                n174 = Unbundle(w290) -> (w286:string[])
                n175 = Match First String(2:w286, 3:w291) -> (0:w287:i32)  [unwired: 1 out]
                n176 = property on="Test Ring" class="Ring (strict)"("Value"=w287, "Strings []"=w286) -> ()  [unwired: 2 in, 2 out]
                n177 = property on="Test Ring" class="Ring (strict)"("Visible"=TRUE) -> ()  [unwired: 2 in, 2 out]
                n178 = property on="Test Slider" class="Slide (strict)"("Visible"=FALSE) -> ()  [unwired: 2 in, 2 out]
              }
              frame "Color Enable  **" {
                n179 = Index Array(array=w298, index=4) -> (element=w299:cluster{string[]})
                n180 = call <vilib>:"NT Read String.vi"("Name"=w301) -> ("String"=w300:string)  [unwired: 9 in, 1 out]
                n181 = Unbundle(w299) -> (w295:string[])
                n182 = Match First String(2:w295, 3:w300) -> (0:w296:i32)  [unwired: 1 out]
                n183 = property on="Test Ring" class="Ring (strict)"("Value"=w296, "Strings []"=w295) -> ()  [unwired: 2 in, 2 out]
                n184 = property on="Test Ring" class="Ring (strict)"("Visible"=TRUE) -> ()  [unwired: 2 in, 2 out]
                n185 = property on="Test Slider" class="Slide (strict)"("Visible"=FALSE) -> ()  [unwired: 2 in, 2 out]
              }
              frame Default {
                n186 = property on="Test Ring" class="Ring (strict)"("Visible"=FALSE) -> ()  [unwired: 2 in, 2 out]
                n187 = property on="Test Slider" class="Slide (strict)"("Visible"=FALSE) -> ()  [unwired: 2 in, 2 out]
              }
              frame "Brightness  **", "Color Level  **", "Compression  **", "FPS  **", "Sharpness  **" {
                n188 = call <vilib>:"NT Read Number.vi"("Name"=w307) -> ("Numeric"=w306:dbl)  [unwired: 9 in, 1 out]
                n189 = local write "Test Slider"(w306) -> ()
                n190 = property on="Test Slider" class="Slide (strict)"("Visible"=TRUE, "Scale.Maximum"=100.0 ("Scale.Range:Maximum")) -> ()  [unwired: 2 in, 2 out]
                n191 = property on="Test Ring" class="Ring (strict)"("Visible"=FALSE) -> ()  [unwired: 2 in, 2 out]
              }
            }
          }
        }
        n192 = property on="Progress" class="Clust (strict)"("Visible"=FALSE) -> ()  [unwired: 2 in, 2 out]
      }
      event "Test Name": Mouse Enter {
        # "Populate the ring with the list of tests"
        n193 = event-data() -> ()  [unwired: 1 in, 1 out]
        n194 = call <vilib>:"NT Read String Array.vi"("Name"="TestMode/TestList") -> ("String Array"=w315:string[])  [unwired: 9 in, 1 out]
        n195 = Build Array (concatenate)("Select the test to run...", w315) -> (w314:string[])
        n196 = property on="Test Name" class="Ring (strict)"("Strings []"=w314) -> ()  [unwired: 2 in, 2 out]
      }
      event "Test Name": Value Change {
        w317 = FALSE ("Visible")
        # "Tell the robot the test name to run"
        n197 = event-data() -> ("NewVal"=w321:u16)  [unwired: 1 in]
        n198 = property on="Test Name" class="Ring (strict)"() -> ("Strings []"=w322:string[])  [unwired: 2 in, 2 out]
        n199 = local write "Progress"(T9 {"Test Progress"=0, "Test Progress Text"=""} ("Progress")) -> ()
        n200 = Index Array(array=w322, index=w321) -> (element=w320:string)
        n201 = call <vilib>:"NT Write String.vi"("String"=w320, "Name"="TestMode/TestName") -> ()  [unwired: 9 in, 1 out]
        n202 = property on="Progress" class="Clust (strict)"("Visible"=TRUE) -> ()  [unwired: 2 in, 2 out]
        n203 = property on="Motor" class="Clust (strict)"("Visible"=w317) -> ()  [unwired: 2 in, 2 out]
        n204 = property on="Test Slider" class="Slide (strict)"("Visible"=w317) -> ()  [unwired: 2 in, 2 out]
        n205 = property on="On/Off" class="Bool (strict)"("Visible"=w317) -> ()  [unwired: 2 in, 2 out]
        n206 = property on="Rev/Fwd" class="Clust (strict)"("Visible"=w317) -> ()  [unwired: 2 in, 2 out]
        n207 = property on="Test Ring" class="Ring (strict)"("Visible"=w317) -> ()  [unwired: 2 in, 2 out]
      }
      event "Listbox": Double Click {
        # "Shift clears all"
        # "Update symbols on the listbox"
        n208 = event-data() -> ("PlatMods.Shift"=w325:bool, "Row"=w327:i32)  [unwired: 1 in]
        n209 = case shown="True" w325 {
          tunnel: w327 -> [w331 _]
          tunnel: 1 -> [w330 _]
          frame False {
            n210 = property on="Listbox" class="LstBox (strict)"() -> ("Item Symbols"=w329:i32[])  [unwired: 2 in, 2 out]
            n211 = Replace Array Subset(array=w329, new element=w330, index=w331) -> (w328:i32[])
            n212 = property on="Listbox" class="LstBox (strict)"("Item Symbols"=w328) -> ()  [unwired: 2 in, 2 out]
          }
          frame True {
            w332 = 0 ("Top Row")
            n213 = property on="Listbox" class="LstBox (strict)"() -> ("Number of Rows"=w334:u32)  [unwired: 2 in, 2 out]
            n214 = Initialize Array(0, w334) -> (w333:i32[])
            n215 = property on="Listbox" class="LstBox (strict)"("Top Row"=w332, "Value"=w332, "Item Symbols"=w333) -> ()  [unwired: 2 in, 2 out]
          }
        }
      }
      event "Listbox": Key Down {
        # "Update symbols on the listbox\nLeft and right keys check and uncheck"
        n216 = event-data() -> ("VKey"=w338:T23)  [unwired: 1 in]
        n217 = case shown="\"Left\", \"Right\"" w338 {
          selector: w338 -> [w343 _]
          tunnel: eventvkey."Left" ("VKey") -> [w341 _]
          frame "Left", "Right" {
            n218 = Equal?(x=w341, y=w343) -> (x = y?=w342:bool)
            n219 = Select(t=0, s=w342, f=1) -> (s? t:f=w344:i32)
            n220 = property on="Listbox" class="LstBox (strict)"() -> ("Item Symbols"=w347:i32[])  [unwired: 2 in, 2 out]
            n221 = Replace Array Subset(array=w347, new element=w344, index="Listbox") -> (w346:i32[])
            n222 = property on="Listbox" class="LstBox (strict)"("Item Symbols"=w346) -> ()  [unwired: 2 in, 2 out]
          }
          frame Default {
          }
        }
      }
      event "DB Camera Config": Value Change {
        # "Show or hide the cluster of controls, store in ini file"
        n223 = event-data() -> ("NewVal"=w351:bool)  [unwired: 1 in]
        n224 = case shown="False" w351 {
          tunnel: w350 -> [w360 _]
          tunnel: [w353 w371] -> w349
          tunnel: w348 -> [w352 w371]
          frame False {
            w367 = "Camera"
            w370 = FALSE ("Visible")
            n225 = local read "Camera Settings"() -> (w359:T2)
            n226 = Index Array(array=w360) -> (element=w363:cluster{string[]})  [unwired: 1 in]
            n227 = Unbundle(w359) -> ("Frame Rate"=w358:i32, "Compression"=w357:i32, "Size"=w361:u16)
            n228 = Unbundle(w363) -> (w362:string[])
            n229 = Index Array(array=w362, index=w361) -> (element=w356:string)
            n230 = call-poly <vilib>:"Write Key.vi"("section"=w367, "value"=w356, "key"="Size", "refnum"=w352) -> ("refnum out"=w369:T21)  [unwired: 2 in, 5 out]
            n231 = call-poly <vilib>:"Write Key.vi"("section"=w367, "value"=w358, "key"="FrameRate", "refnum"=w369) -> ("refnum out"=w368:T21)  [unwired: 1 in, 6 out]
            n232 = property on="Camera Settings" class="Clust (strict)"("Visible"=w370) -> ()  [unwired: 2 in, 2 out]
            n233 = local write "DB Camera Config"(w370) -> ()
            n234 = call-poly <vilib>:"Write Key.vi"("section"=w367, "value"=w357, "key"="Compression", "refnum"=w368) -> ("refnum out"=w354:T21)  [unwired: 1 in, 6 out]
            n235 = call <vilib>:"Close Config Data.vi"("refnum"=w354) -> ("file path"=w355:path)  [unwired: 2 in, 8 out]
            n236 = call <vilib>:"Open Config Data.vi"("configuration file path"=w355) -> ("refnum"=w353:T21)  [unwired: 8 in, 2 out]
          }
          frame True {
            n237 = property on="Camera Settings" class="Clust (strict)"("Visible"=TRUE) -> ()  [unwired: 2 in, 2 out]
          }
        }
      }
      event "Camera Settings": Value Change {
        # "Update summary string when any elements of DB camera change"
        n238 = event-data() -> ("NewVal"=w384:T2)  [unwired: 1 in]
        n239 = Index Array(array=w380) -> (element=w379:cluster{string[]})  [unwired: 1 in]
        n240 = Unbundle(w384) -> ("Frame Rate"=w375:i32, "Compression"=w374:i32, "Size"=w377:u16)
        n241 = Unbundle(w379) -> (w378:string[])
        n242 = Index Array(array=w378, index=w377) -> (element=w376:string)
        n243 = Format Into String(format string="%s   %dfps   %d%%", w376, w375, w374) -> (resulting string=w381:string)  [unwired: 2 in, 1 out]
        n244 = Build Array(w381) -> (w382:string[])
        n245 = property on="DB Camera Config" class="Bool (strict)"("Strings [4]"=w382) -> ()  [unwired: 2 in, 2 out]
      }
      event "Motor.Enable": Value Change {
        # "When the test mode otor enable helper is set, update that\ntree row item's value"
        n246 = event-data() -> ("NewVal"=w390:bool)  [unwired: 1 in]
        n247 = Unbundle("Motor") -> ("Value"=w389:dbl)  [unwired: 1 out]
        n248 = Select(t=w389, s=w390, f=0.0) -> (s? t:f=w387:dbl)
        n249 = call <vilib>:"NT Write Number.vi"("Numeric"=w387, "Name"=w386) -> ()  [unwired: 9 in, 1 out]
      }
      event "Test Slider": Value Change {
        # "When the test mode slider helper is set, update that\ntree row item's value"
        n250 = event-data() -> ("NewVal"=w393:dbl)  [unwired: 1 in]
        n251 = call <vilib>:"NT Write Number.vi"("Numeric"=w393, "Name"=w394) -> ()  [unwired: 9 in, 1 out]
      }
      event "On/Off": Value Change {
        # "When the test mode on/off helper value is set, update that\ntree row item's value"
        n252 = event-data() -> ("NewVal"=w398:bool)  [unwired: 1 in]
        n253 = Boolean To (0,1)(Boolean=w398) -> (0, 1=w397:i16)
        n254 = call <vilib>:"NT Write Number.vi"("Numeric"=w397, "Name"=w396) -> ()  [unwired: 9 in, 1 out]
      }
      event "Rev/Fwd": Value Change {
        # "When the test mode helper value for relays is set, update that\ntree row item's value"
        n255 = event-data() -> ("NewVal.Forward"=w406:bool, "NewVal.Reverse"=w405:bool)  [unwired: 1 in]
        n256 = Boolean To (0,1)(Boolean=w406) -> (0, 1=w402:i16)
        n257 = Boolean To (0,1)(Boolean=w405) -> (0, 1=w404:i16)
        n258 = Negate(x=w404) -> (-x=w403:i16)
        n259 = Add(x=w402, y=w403) -> (x+y=w401:i16)
        n260 = call <vilib>:"NT Write Number.vi"("Numeric"=w401, "Name"=w400) -> ()  [unwired: 9 in, 1 out]
      }
      event "Test Ring": Value Change {
        # "When a test mode helper value is selected from the ring,\nset the tree item's variable to the string value"
        n261 = event-data() -> ("NewVal"=w410:u16)  [unwired: 1 in]
        n262 = property on="Test Ring" class="Ring (strict)"() -> ("Strings []"=w411:string[])  [unwired: 2 in, 2 out]
        n263 = Index Array(array=w411, index=w410) -> (element=w409:string)
        n264 = call <vilib>:"NT Write String.vi"("String"=w409, "Name"=w408) -> ()  [unwired: 9 in, 1 out]
      }
      event "Rec Mode": Value Change {
        # "Update globals for recording mode and path to read log from.\nClear when logging and let NetworkTables set path for vision to\nuse."
        n265 = event-data() -> ("NewVal"=w421:enum32{"Stop", "Record", "Playback"})  [unwired: 1 in]
        n266 = global write "WPI_DashboardLogging Global.vi" "Logging Filename"(path "") -> ()
        n267 = case shown="\"Playback\"" w421 {
          tunnel: w420 -> [_ w423 w431]
          tunnel: [_ _ w430] -> w417
          tunnel: [_ _ w429] -> _
          tunnel: w415 -> [_ _ w427]
          tunnel: cluster{i32, i32} {-250, 170} -> [_ _ w426]
          tunnel: [_ _ T24 {"Image Size"=TRUE, "Image Type"=TRUE, "Pixel Value"=TRUE, "ROI Information"=TRUE, "Zoom Factor"=FALSE} ("Image Information Shown:All Elements")] -> w413
          tunnel: [_ _ TRUE ("Zoom Factor")] -> w412
          frame Default {
          }
          frame "Stop", "Record" {
            # "Place Window too"
            n268 = invoke class="VI" method="FP.Close"(reference=w423) -> (reference out=w422:refnum<vi>)  [unwired: 2 in, 2 out]
            n269 = invoke class="VI" method="Abort VI"(reference=w422) -> ()  [unwired: 2 in, 3 out]
          }
          frame "Playback" {
            n270 = call "Open Playback Panel.vi"("Offset"=w426, "DB VI Ref"=w427, "Playback in"=w431) -> ("Playback out"=w428:refnum<vi>)  [unwired: 8 in]
            n271 = register-events(w428) -> (reference out=w430:refnum<event-registration>, error out=w429:errorcluster)  [unwired: 2 in]
          }
        }
        n272 = global write "WPI_DashboardLogging Global.vi" "Recording"(w421) -> ()
        n273 = property on="Camera Image" class="ImageControl"("Image Information Shown"=w413, "Image Information Visible"=w412) -> ()  [unwired: 2 in, 2 out]
        n274 = call <vilib>:"WPI_DashboardNT Log FieldName Cache.vi"("Operation"=enum16{"Lookup/Add", "Index", "Clear"}."Clear") -> ()  [unwired: 8 in, 3 out]
      }
      event Panel Close {
        w432 = enum32{"Stop", "Record", "Playback"}."Stop" ("Rec Mode")
        # "Playback window has been closed, abort"
        n275 = event-data() -> ()  [unwired: 1 in, 4 out]
        n276 = local write "Rec Mode"(w432) -> ()
        n277 = global write "WPI_DashboardLogging Global.vi" "Recording"(w432) -> ()
      }
      event Panel Close {
        # "Abort playback window and ourself"
        n278 = event-data() -> ()  [unwired: 1 in, 4 out]
        n279 = invoke class="VI" method="FP.Close"(reference=w437) -> (reference out=w436:refnum<vi>)  [unwired: 2 in, 2 out]
        n280 = invoke class="VI" method="Abort VI"(reference=w436) -> (error out=w435:errorcluster)  [unwired: 2 in, 2 out]
        n281 = invoke class="VI" method="Abort VI"(error in=w435) -> ()  [unwired: 2 in, 3 out]
      }
      event "Vision": Value Change {
        # "Enable/Disable Compression slider.\nHW USB is hard-coded into the camera"
        n282 = event-data() -> ("NewVal"=w443:u16)  [unwired: 1 in]
        n283 = Equal?(x=w443, y=u32 2 ("milliseconds to wait")) -> (x = y?=w441:bool)
        n284 = Select(t=T25."Disabled and Grayed Out" ("Disabled"), s=w441, f=T25."Enabled" ("Disabled")) -> (s? t:f=w438:T25)
        n285 = property on="Compression" class="Slide (strict)"("DisabledEnum"=w438) -> ()  [unwired: 2 in, 2 out]
      }
    }
  }
  n286 = while {
    tunnel: w38 -> [w446]
    i -> [w449]
    stop <- FALSE stop-if-true
    n287 = Wait (ms)(milliseconds to wait=u32 100) -> ()  [unwired: 1 out]
    n288 = case shown="\"Playback\"" "Rec Mode" {
      tunnel: w449 -> [_ _ w464]
      tunnel: [u32 2829099 ("Base Color") u32 11141120 ("Target Color") w453] -> w445
      frame "Stop", Default {
        # "Reset the color, extra updates don't cost much"
      }
      frame "Record" {
      }
      frame "Playback" {
        # "Playback"
        n289 = Quotient & Remainder(x=w464, y=u32 50 ("milliseconds to wait")) -> (x-y*floor(x/y)=w460:u32)  [unwired: 1 out]
        n290 = Divide(x=w460, y=u32 50 ("milliseconds to wait")) -> (x/y=w457:dbl)
        n291 = Multiply(x=6.283185307179586, y=w457) -> (x*y=w462:dbl)
        n292 = Sine(x=w462) -> (sin(x)=w461:dbl)
        n293 = Absolute Value(x=w461) -> (abs(x)=w454:dbl)
        n294 = call "Interpolate RGB Color.vi"("Proportion"=w454, "Target Color"=u32 30976, "Base Color"=u32 2829099) -> ("Result Color"=w453:u32)  [unwired: 8 in]
      }
    }
    n295 = property class="Pane"(reference=w446, "PaneColor"=w445) -> ()  [unwired: 1 in, 2 out]
  }
  n296 = TCP Create Listener(10:u16 1741 ("timeout ms (25000)")) -> (3:w1:refnum<k5>)  [unwired: 4 in, 2 out]
  n297 = while {
    tunnel: w1 -> [w466]
    stop <- FALSE stop-if-true
    n298 = TCP Wait On Listener(11:w466) -> (4:w465:refnum<k5>)  [unwired: 3 in, 4 out]
    n299 = local write "TCP"(w465) -> ()
  }
  n300 = property on="On/Off" class="Bool (strict)"("Visible"=w6) -> ()  [unwired: 2 in, 2 out]
  n301 = property on="Motor" class="Clust (strict)"("Visible"=w6) -> ()  [unwired: 2 in, 2 out]
  n302 = property on="Progress" class="Clust (strict)"("Visible"=w6) -> ()  [unwired: 2 in, 2 out]
  n303 = property on="Test Ring" class="Ring (strict)"("Visible"=w6) -> ()  [unwired: 2 in, 2 out]
  n304 = property on="Rev/Fwd" class="Clust (strict)"("Visible"=w6) -> ()  [unwired: 2 in, 2 out]
  n305 = property on="Camera Settings" class="Clust (strict)"("Visible"=w6) -> ()  [unwired: 2 in, 2 out]
  n306 = local write "DB Camera Config"(w6) -> ()
  n307 = global write "WPI_DashboardLogging Global.vi" "Recording"(w32) -> ()
  n308 = local write "Rec Mode"(w32) -> ()
